vi "NInstrSim.Main.vi"() -> ()   [LabVIEW 2009, in "HB_Device_Examples.lvlib"]
doc: "Simple demo VI."
uses:
  HB_Device_Examples.lvlib
  NInstrSim/Factory/HB_DeviceFactory.lvclass
  NInstrSim/NInstrSim.lvclass
  lib.lib/HGF_LVC/HGF_BaseClasses/HGF_Notifier/HGF_Notifier.lvclass
  lib.lib/HGF_LVC/HGF_BaseClasses/HGF_Factory/HGF_Factory.lvclass
  lib.lib/HGF_LVC/HGF_Auxiliary/HGF_Auxiliary.lvlib
  lib.lib/HGF_LVC/HGF_DeviceBaseClasses/HGF_VISADevice/HGF_VISADevice.lvclass
  lib.lib/HGF_LVC/HGF_DeviceBaseClasses/HGF_DeviceBase/HGF_DeviceBase.lvclass
  lib.lib/HGF_LVC/HGF_BaseClasses/HGF_Event/HGF_Event.lvclass
panel:
  in  "timeout in ms (-1)":i32=3000
  in  "Byte Order (0:Low Byte First)":u16(ring) items=["Low Byte First", "High Byte First"]
  in  "Waveform Format (0:ASCII)":u16(ring) items=["ASCII", "8-bit Unsigned Binary", "16-bit Signed Binary"]
  out "Waveform Graph":waveform(dbl)(graph)
  out "DC Measurement":dbl format="%_6g"
  in  "DC Voltage Range (1:10 VDC)":u16(ring)=1 items=["0:1 VDC", "0:10 VDC", "0:100 VDC"]
  in  "stop":bool
  out "model":string="unknown"
  out "vendor":string="unknown"
  out "firmwareRevision":string="unknown"
  out "driverRevision":string="unknown"
  out "passed?":bool
  in  "Serial Configuration":T1={"Baud Rate"=9600, "Flow Control"=0, "Parity"=0, "Data Bits"=7, "Stop Bits"=10} {"Stop Bits" items=["1.0"=10, "1.5"=15, "2.0"=20]; "Data Bits" items=["7"=7, "8"=8]; "Parity" items=["None", "Odd", "Even", "Mark", "Space"]; "Flow Control" items=["None"=0, "XON/XOFF"=1, "RTS/CTS"=2, "DTR/DSR"=4]; "Baud Rate" items=["300"=300, "600"=600, "1200"=1200, "2400"=2400, "4800"=4800, "9600"=9600, "19200"=19200]}
  in  "VISA Resource Name":refnum<visa-resource-name>
  in  "objectName":string
  out "initData found?":bool
  in  "Use Factory?":bool
  out "className":string
  out "objectName":string
  out "initialized?":bool
  out "createdFromFactory?":bool
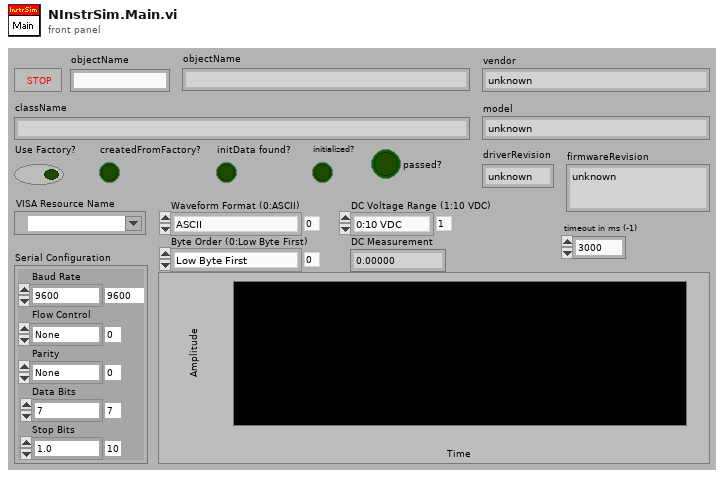
[diagram p1: front panel]
types:
  T1 = cluster{"Baud Rate":u32, "Flow Control":u16, "Parity":u16, "Data Bits":u16, "Stop Bits":u16}
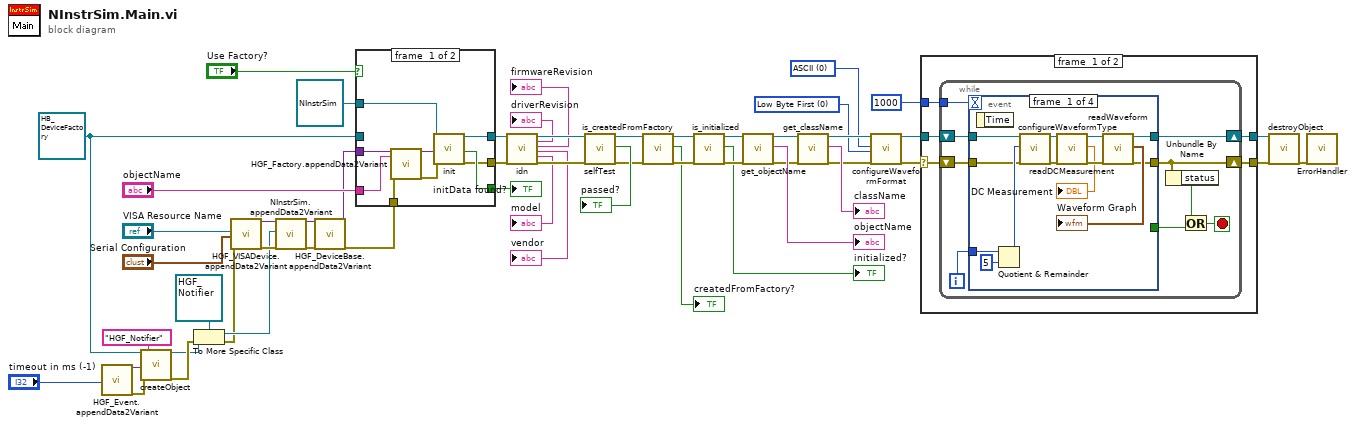
[diagram p0: block diagram]
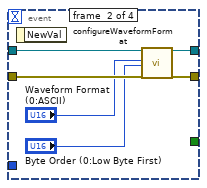
[diagram p2: hidden frame]
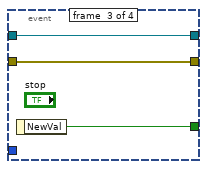
[diagram p3: hidden frame]
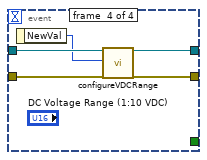
[diagram p4: hidden frame]
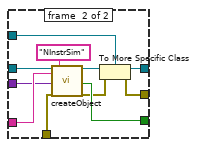
[diagram p6: hidden frame]
diagram:
  w23 = u16 0 items=["Low Byte First", "High Byte First"] ("Byte Order (0:Low Byte First)")
  w24 = u16 0 items=["ASCII", "8-bit Unsigned Binary", "16-bit Signed Binary"] ("Waveform Format (0:ASCII)")
  w1 = refnum<class "HB_DeviceFactory.lvclass"> refnum ("HB_Device_Examples.lvlib:HB_DeviceFactory.lvclass")
  n1 = call "HGF_Event.appendData2Variant.vi"("timeout in ms (-1)"="timeout in ms (-1)") -> ("dup initData"=w8:variant, "error out"=w9:errorcluster)  [unwired: 2 in, 15 out]
  n2 = call "createObject.vi"("HGF_Factory"=w1, "initializationData"=w8, "error in (no error)"=w9, "className"="HGF_Notifier") -> ("HGF_Object"=w5:refnum<class "HGF_Factory.lvclass">, "error out"=w6:errorcluster)  [unwired: 2 in, 12 out]
  n3 = To More Specific Class(target class=refnum<class "HGF_Notifier.lvclass"> refnum ("HGF_BaseClasses.lvlib:HGF_Notifier.lvclass"), reference=w5, error in=w6) -> (specific class reference=w3:refnum<class "HGF_Notifier.lvclass">, error out=w2:errorcluster)
  n4 = call "HGF_VISADevice.appendData2Variant.vi"("VISA Resource Name"="VISA Resource Name", "Serial Configuration"="Serial Configuration", "error in (no error)"=w2) -> ("dup initData"=w14:variant, "error out"=w12:errorcluster)  [unwired: 1 in, 14 out]
  n5 = call "NInstrSim.appendData2Variant.vi"("initData"=w14, "statusEvent"=w3, "error in (no error)"=w12) -> ("dup initData"=w13:variant, "error out"=w11:errorcluster)  [unwired: 15 out]
  n6 = call "HGF_DeviceBase.appendData2Variant.vi"("initData"=w13, "error in (no error)"=w11) -> ("dup initData"=w40:variant, "error out"=w39:errorcluster)  [unwired: 16 out]
  n7 = case shown="True" "Use Factory?" {
    tunnel: [w62 w71] -> w22
    tunnel: [w60 w68] -> w21
    tunnel: refnum<class "NInstrSim.lvclass"> refnum ("HB_HGF_Test.lvlib:NInstrSim.lvclass") -> [w57 w69]
    tunnel: [w61 w72] -> w43
    tunnel: w1 -> [_ w67]
    tunnel: "objectName" -> [w54 w66]
    tunnel: w40 -> [w56 w64]
    tunnel: w39 -> [w55 w63]
    frame #0 {
      n8 = call "HGF_Factory.appendData2Variant.vi"("initData"=w56, "objectName"=w54, "error in (no error)"=w55) -> ("dup initData"=w58:variant, "error out"=w59:errorcluster)  [unwired: 2 in, 13 out]
      n9 = call "init.vi"("HGF_Object"=w57, "initializationData"=w58, "error in (no error)"=w59) -> ("dup HGF_Object"=w62:refnum<class "NInstrSim.lvclass">, "found?"=w61:bool, "error out"=w60:errorcluster)  [unwired: 14 out]
    }
    frame #1 {
      n10 = call "createObject.vi"("HGF_Factory"=w67, "objectName"=w66, "initializationData"=w64, "error in (no error)"=w63, "className"="NInstrSim") -> ("HGF_Object"=w65:refnum<class "HGF_Factory.lvclass">, "found?"=w72:bool, "error out"=w70:errorcluster)  [unwired: 12 out]
      n11 = To More Specific Class(target class=w69, reference=w65, error in=w70) -> (specific class reference=w71:refnum<class "NInstrSim.lvclass">, error out=w68:errorcluster)
    }
  }
  "initData found?" <- w43
  n12 = call "idn.vi"("HGF_DeviceBase"=w22, "error in (no error)"=w21) -> ("dup HGF_DeviceBase"=w20:refnum<class "NInstrSim.lvclass">, "driverRevision"=→"driverRevision":string, "firmwareRevision"=→"firmwareRevision":string, "vendor"=→"vendor":string, "model"=→"model":string, "error out"=w19:errorcluster)  [unwired: 8 in, 4 out]
  n13 = call-dynamic "selfTest.vi"("NInstrSim"=w20, "error in (no error)"=w19) -> ("dup NInstrSim"=w35:refnum<class "NInstrSim.lvclass">, "passed?"=→"passed?":bool, "error out"=w34:errorcluster)  [unwired: 15 out]
  n14 = call "is_createdFromFactory.vi"("HGF_Factory"=w35, "error in (no error)"=w34) -> ("dup HGF_Factory"=w30:refnum<class "NInstrSim.lvclass">, "createdFromFactory?"=→"createdFromFactory?":bool, "error out"=w53:errorcluster)  [unwired: 15 out]
  n15 = call "is_initialized.vi"("HGF_Factory"=w30, "error in (no error)"=w53) -> ("dup HGF_Factory"=w52:refnum<class "NInstrSim.lvclass">, "initialized?"=→"initialized?":bool, "error out"=w51:errorcluster)  [unwired: 15 out]
  n16 = call "get_objectName.vi"("HGF_Factory"=w52, "error in (no error)"=w51) -> ("dup HGF_Factory"=w47:refnum<class "NInstrSim.lvclass">, "objectName"=→"objectName":string, "error out"=w46:errorcluster)  [unwired: 15 out]
  n17 = call "get_className.vi"("HGF_Factory"=w47, "error in (no error)"=w46) -> ("dup HGF_Factory"=w28:refnum<class "NInstrSim.lvclass">, "className"=→"className":string, "error out"=w25:errorcluster)  [unwired: 15 out]
  n18 = call "configureWaveformFormat.vi"("NInstrSim"=w28, "Waveform Format (0:ASCII)"=w24, "Byte Order (0:Low Byte First)"=w23, "error in (no error)"=w25) -> ("dup NInstrSim"=w27:refnum<class "NInstrSim.lvclass">, "error out"=w26:errorcluster)  [unwired: 14 out]
  n19 = case shown="No Error" w26 {
    selector: w26 -> [w77 w116]
    tunnel: [w75 w116] -> w33
    tunnel: w27 -> [w78 w115]
    tunnel: [w76 w115] -> w31
    tunnel: 1000 -> [w74 _]
    frame #0 {
      n20 = while {
        shift-right: [w85] -> w76
        shift-left: w78 -> [w87]
        shift-right: [w82] -> w75
        shift-left: w77 -> [w86]
        tunnel: w74 -> [w80]
        i -> [w79]
        stop <- w83 stop-if-true
        n21 = event shown="[2] \"stop\": Value Change" {
          selector: _ -> [_ _ _ _]
          dyn-events: _ -> [_ _ _ _]
          timeout: w80 -> [_ _ _ _]
          tunnel: w87 -> [w91 w106 w107 w114]
          tunnel: w86 -> [w90 w104 w109 w113]
          tunnel: [w93 w105 w107 w111] -> w85
          tunnel: [w92 w103 w109 w110] -> w82
          tunnel: [_ _ w108 _] -> w84
          tunnel: w79 -> [w96 _ _ _]
          event #0 {
            n22 = event-data() -> ()  [unwired: 2 out]
            n23 = Quotient & Remainder(x=w96, y=5) -> (x-y*floor(x/y)=w94:i32)  [unwired: 1 out]
            n24 = call "configureWaveformType.vi"("NInstrSim"=w91, "function (0:Sine)"=w94, "error in (no error)"=w90) -> ("dup NInstrSim"=w89:refnum<class "NInstrSim.lvclass">, "error out"=w88:errorcluster)  [unwired: 15 out]
            n25 = call "readDCMeasurement.vi"("NInstrSim"=w89, "error in (no error)"=w88) -> ("dup NInstrSim"=w100:refnum<class "NInstrSim.lvclass">, "DC Measurement"=→"DC Measurement":dbl, "error out"=w99:errorcluster)  [unwired: 15 out]
            n26 = call "readWaveform.vi"("NInstrSim"=w100, "error in (no error)"=w99) -> ("dup NInstrSim"=w93:refnum<class "NInstrSim.lvclass">, "Waveform"=→"Waveform Graph":waveform(dbl), "error out"=w92:errorcluster)  [unwired: 15 out]
          }
          event #1 {
            n27 = event-data() -> ()  [unwired: 2 out]
            n28 = call "configureWaveformFormat.vi"("NInstrSim"=w106, "Waveform Format (0:ASCII)"="Waveform Format (0:ASCII)", "Byte Order (0:Low Byte First)"="Byte Order (0:Low Byte First)", "error in (no error)"=w104) -> ("dup NInstrSim"=w105:refnum<class "NInstrSim.lvclass">, "error out"=w103:errorcluster)  [unwired: 14 out]
          }
          event #2 {
            n29 = event-data() -> ("NewVal"=w108:bool)  [unwired: 1 out]
          }
          event #3 {
            n30 = event-data() -> ("NewVal"=w112:u16)  [unwired: 1 out]
            n31 = call "configureVDCRange.vi"("NInstrSim"=w114, "DC Voltage Range (1:10 VDC)"=w112, "error in (no error)"=w113) -> ("dup NInstrSim"=w111:refnum<class "NInstrSim.lvclass">, "error out"=w110:errorcluster)  [unwired: 15 out]
          }
        }
        n32 = Unbundle By Name(w82) -> ("status"=w81:bool)
        n33 = Or(x=w81, y=w84) -> (x .or. y?=w83:bool)
      }
    }
    frame #1 {
    }
  }
  n34 = call "destroyObject.vi"("HGF_Factory"=w31, "error in (no error)"=w33) -> ("error out"=w32:errorcluster)  [unwired: 17 out]
  n35 = call "ErrorHandler.vi"("error in (no error)"=w32) -> ()  [unwired: 6 in, 13 out]
